vi "Temperature control panel.vi"(8 "error in (no error)":errorcluster, 9 "Data Source (0:Kelvin)":u16(ring) items=["Kelvin", "Celsius", "Sensor Units"], 10 "Input (0:A)":u16(ring) items=["A", "B"], 11 "VISA resource name":refnum<visa-resource-name>="GPIB0::12::INSTR") -> (0 "error out":errorcluster, 2 "Sensor Data":dbl format="%.4f", 3 "VISA resource name out":refnum<visa-resource-name>)   [LabVIEW 2020]
doc: "Reads and returns a single sensor reading from the instrument."
uses:
  Instance           1 36Saved   Sensor Data (Single Reading) .vi
  Lake Shore 335/Lake Shore 335.lvlib
panel:
  in  "Temperature Interval":dbl
  out "Graph":dbl(graph)
  in  "On/Off":bool
  in  "Range (0:Off)":u16(ring) items=["Off", "Low (On)", "Medium", "High"]
  in  "Manual Output (0.00 %)":dbl format="%.2f"
  in  "Heater Output (1:1)":u16(ring)=1 items=["1"=1, "2"=2]
  out "error out 4":errorcluster
  out "VISA resource name out 4":refnum<visa-resource-name>
  in  "error in (no error) 4":errorcluster
  in  "Setpoint start":bool
  in  "error in (no error) 3":errorcluster
  out "VISA resource name out 3":refnum<visa-resource-name>
  out "error out 3":errorcluster
  out "Setpoint":dbl format="%.4f"
  in  "Output (1:1)":u16(ring)=1 items=["1"=1, "2"=2]
  in  "error in (no error) 2":errorcluster
  out "VISA resource name out 2":refnum<visa-resource-name>
  out "error out 2":errorcluster
  in  "Output's Control Loop (1:1)":u16(ring)=1 items=["1"=1, "2"=2]
  in  "Setpoint (0.0000)":dbl format="%.4f"
  in  "Enable Setpoint Ramping (F: Off)":bool
  in  "Ramp Rate (0.0)":dbl=10.0 format="%.1f"
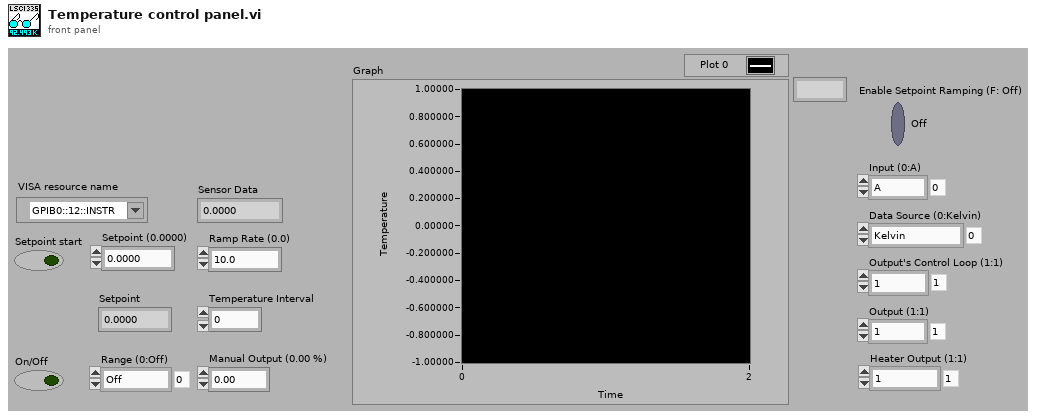
[diagram p1: front panel]
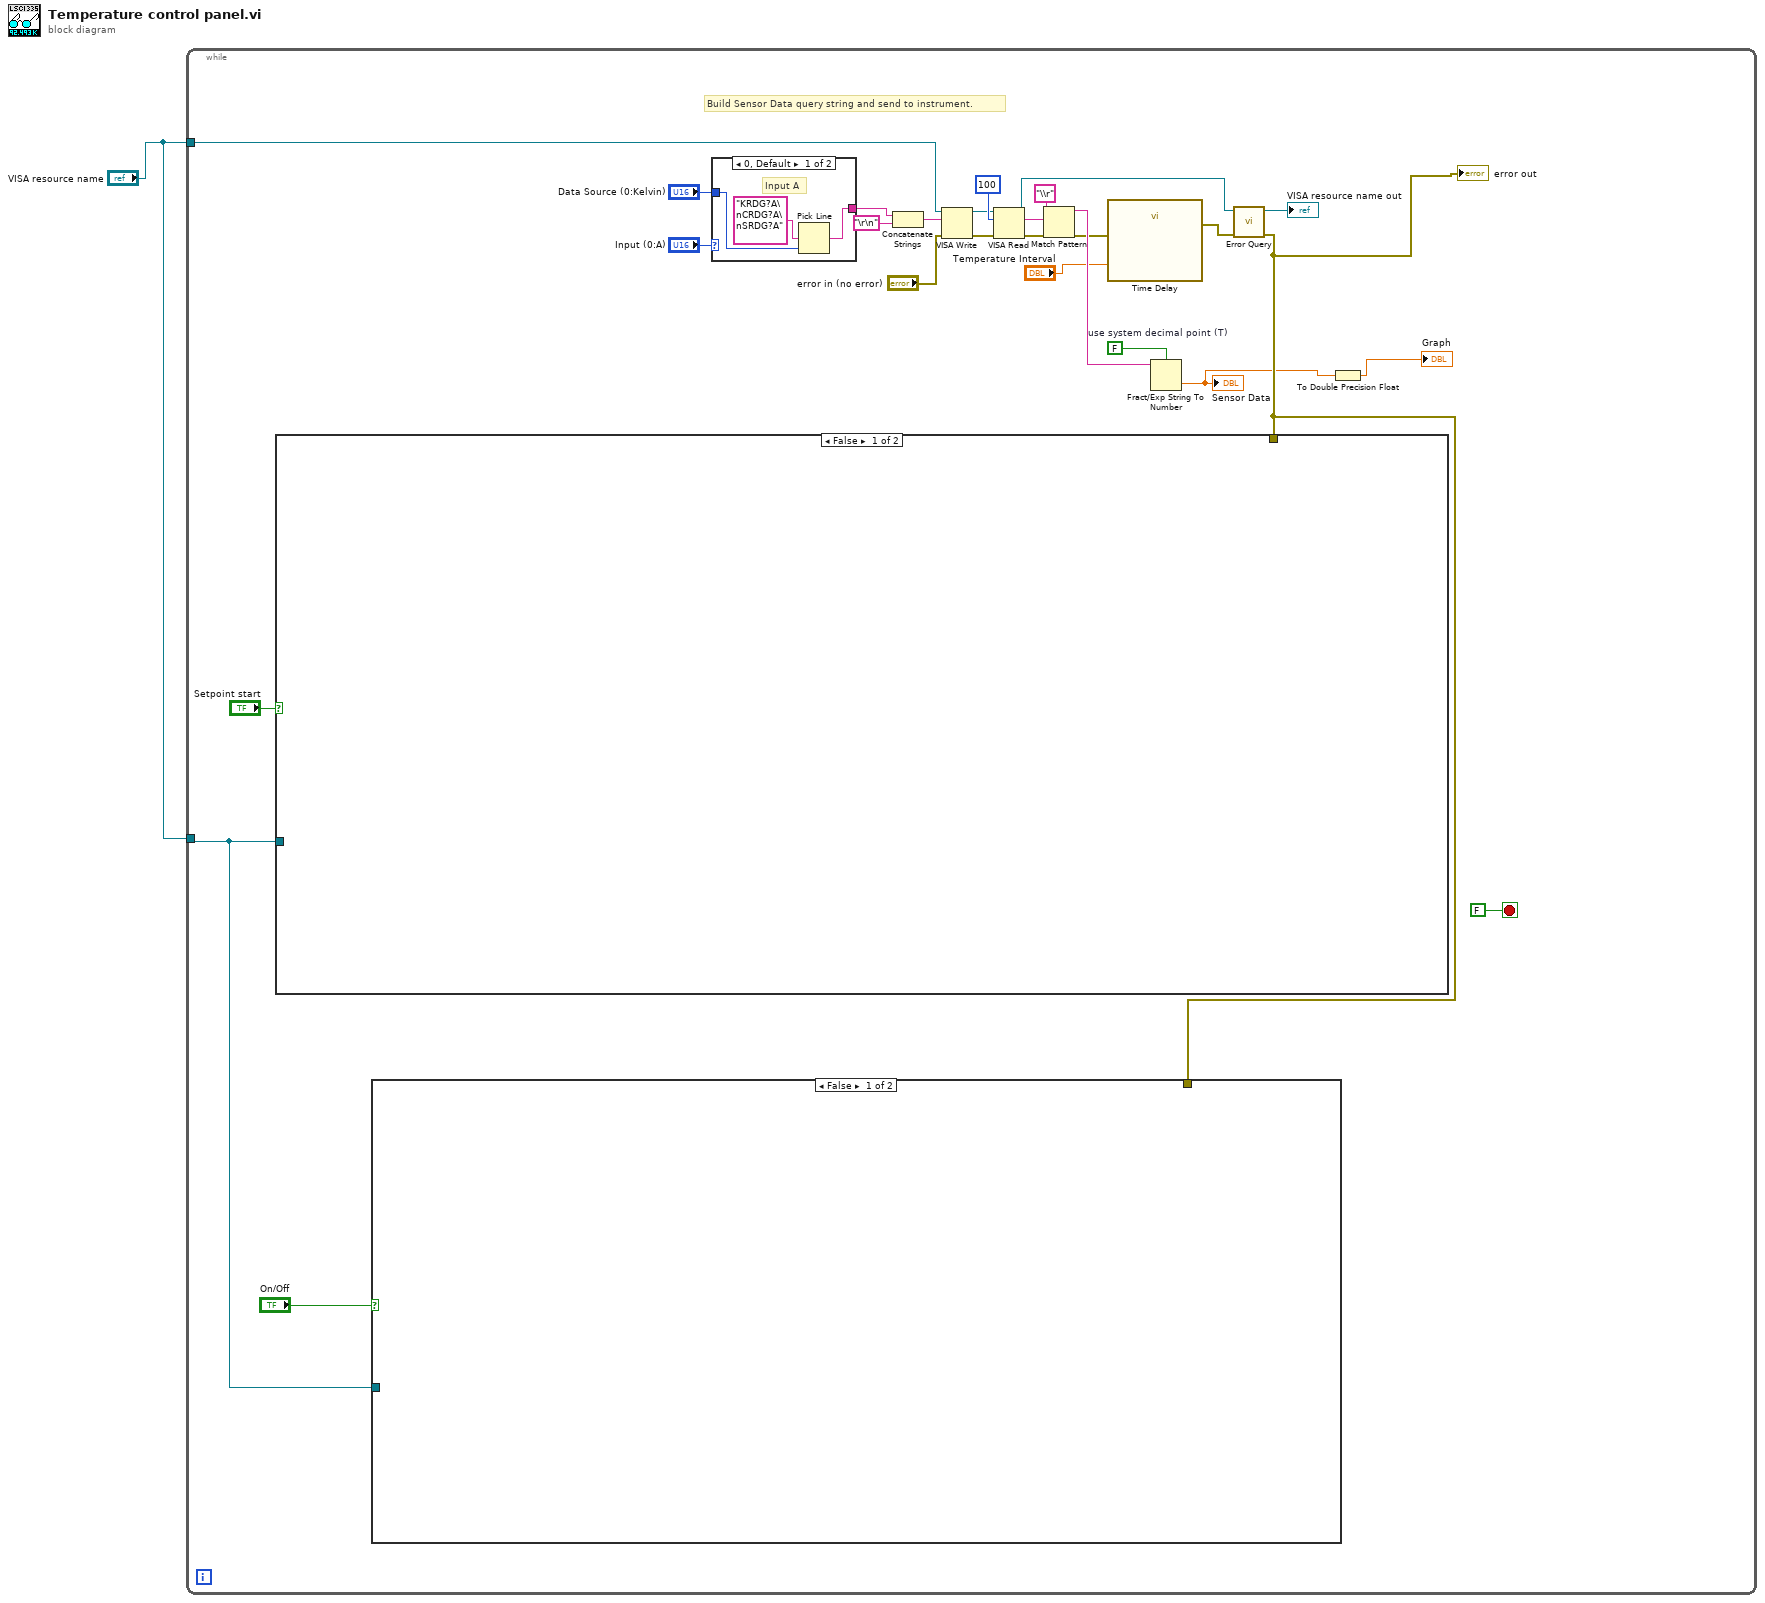
[diagram p0: block diagram]
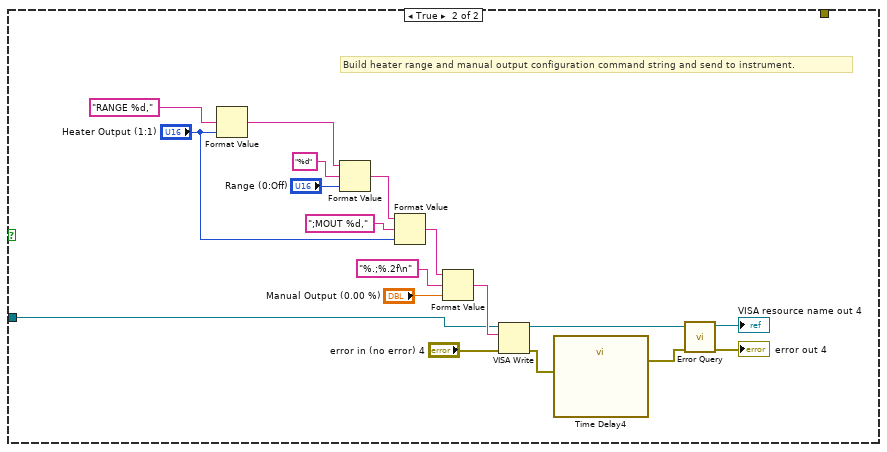
[diagram p2: hidden frame]
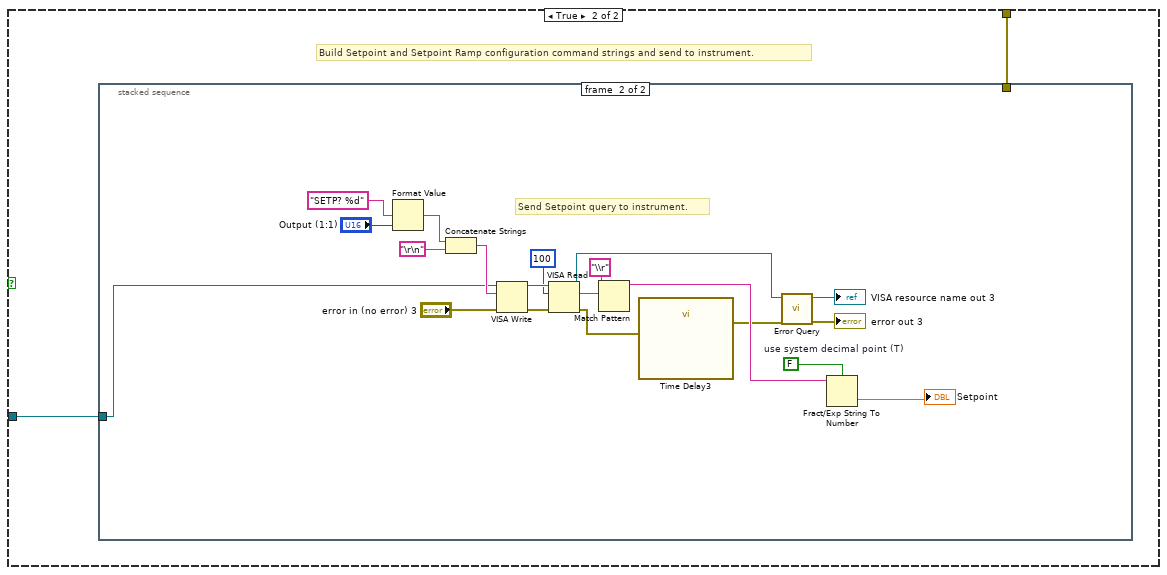
[diagram p3: hidden frame]
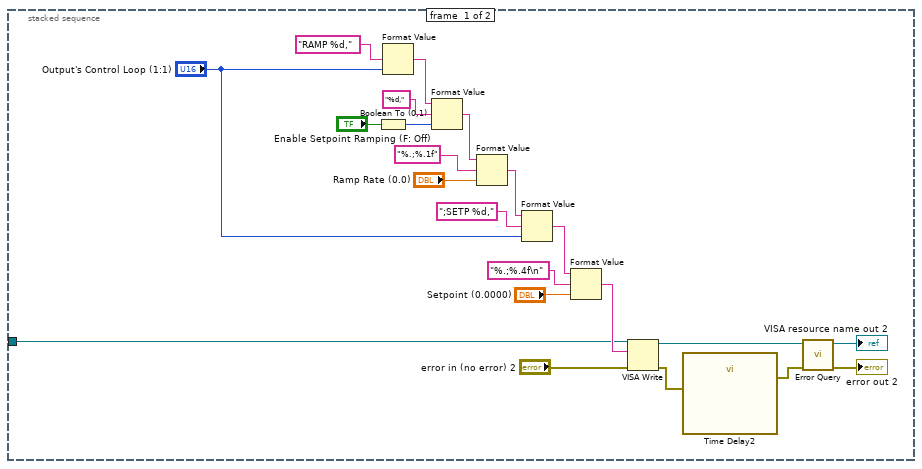
[diagram p4: hidden frame]
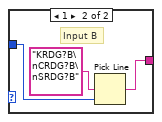
[diagram p5: hidden frame]
diagram:
  n1 = while {
    tunnel: "VISA resource name" -> [w8]
    tunnel: "VISA resource name" -> [w7]
    stop <- FALSE stop-if-true
    w19 = FALSE  # use system decimal point (T)
    # "Build Sensor Data query string and send to instrument."
    n2 = case shown="0, Default" "Input (0:A)" {
      tunnel: "Data Source (0:Kelvin)" -> [w91 w93]
      tunnel: [w90 w94] -> w11
      frame 0, Default {
        # "Input A"
        n3 = Pick Line(multi-line string="KRDG?A\nCRDG?A\nSRDG?A", line index=w91) -> (output string=w90:string)  [unwired: 1 in]
      }
      frame 1 {
        # "Input B"
        n4 = Pick Line(multi-line string="KRDG?B\nCRDG?B\nSRDG?B", line index=w93) -> (output string=w94:string)  [unwired: 1 in]
      }
    }
    n5 = Concatenate Strings(w11, "\r\n") -> (w12:string)
    n6 = VISA Write(VISA resource name=w8, write buffer=w12, error in (no error)="error in (no error)") -> (VISA resource name out=w21:refnum<visa-resource-name>, error out=w20:errorcluster)  [unwired: 1 out]
    n7 = VISA Read(VISA resource name=w21, byte count=100, error in (no error)=w20) -> (VISA resource name out=w25:refnum<visa-resource-name>, read buffer=w23:string, error out=w15:errorcluster)  [unwired: 1 out]
    n8 = Match Pattern(string=w23, regular expression="\\r") -> (before substring=w18:string)  [unwired: 1 in, 3 out]
    n9 = call "Time Delay"("error in (no error)"=w15, "Delay Time (s)"="Temperature Interval") -> ("error out"=w16:errorcluster)  [unwired: 9 in]
    n10 = Fract/Exp String To Number(use system decimal point (T)=w19, string=w18) -> (number=w3:dbl)  [unwired: 2 in, 1 out]
    "Sensor Data" <- w3
    n11 = call "Error Query.vi"("error in (no error)"=w16, "VISA resource name"=w25) -> ("error out"=w5:errorcluster, "VISA resource name out"=→"VISA resource name out":refnum<visa-resource-name>)  [unwired: 7 in, 1 out]
    "error out" <- w5
    n12 = case shown="False" "Setpoint start" {
      tunnel: w5 -> [_ w47]
      tunnel: w7 -> [_ w46]
      frame False {
      }
      frame True {
        # "Build Setpoint and Setpoint Ramp configuration command strings and send to instrument."
        n13 = stacked-sequence {
          tunnel: w47 -> [_ _]
          tunnel: w46 -> [w48 w70]
          frame #0 {
            n14 = Boolean To (0,1)(Boolean="Enable Setpoint Ramping (F: Off)") -> (0, 1=w53:i16)
            n15 = Format Value(format string="RAMP %d,", value (0)="Output's Control Loop (1:1)") -> (output string=w59:string)  [unwired: 1 in]
            n16 = Format Value(string ("")=w59, format string="%d,", value (0)=w53) -> (output string=w55:string)
            n17 = Format Value(string ("")=w55, format string="%.;%.1f", value (0)="Ramp Rate (0.0)") -> (output string=w51:string)
            n18 = Format Value(string ("")=w51, format string=";SETP %d,", value (0)="Output's Control Loop (1:1)") -> (output string=w60:string)
            n19 = Format Value(string ("")=w60, format string="%.;%.4f\n", value (0)="Setpoint (0.0000)") -> (output string=w62:string)
            n20 = VISA Write(VISA resource name=w48, write buffer=w62, error in (no error)="error in (no error) 2") -> (VISA resource name out=w69:refnum<visa-resource-name>, error out=w66:errorcluster)  [unwired: 1 out]
            n21 = call "Time Delay2"("error in (no error)"=w66) -> ("error out"=w65:errorcluster)  [unwired: 10 in]
            n22 = call "Error Query.vi"("error in (no error)"=w65, "VISA resource name"=w69) -> ("error out"=→"error out 2":errorcluster, "VISA resource name out"=→"VISA resource name out 2":refnum<visa-resource-name>)  [unwired: 7 in, 1 out]
          }
          frame #1 {
            w71 = FALSE  # use system decimal point (T)
            # "Send Setpoint query to instrument."
            n23 = Format Value(format string="SETP? %d", value (0)="Output (1:1)") -> (output string=w89:string)  [unwired: 1 in]
            n24 = Concatenate Strings(w89, "\r\n") -> (w81:string)
            n25 = VISA Write(VISA resource name=w70, write buffer=w81, error in (no error)="error in (no error) 3") -> (VISA resource name out=w77:refnum<visa-resource-name>, error out=w78:errorcluster)  [unwired: 1 out]
            n26 = VISA Read(VISA resource name=w77, byte count=100, error in (no error)=w78) -> (VISA resource name out=w84:refnum<visa-resource-name>, read buffer=w75:string, error out=w79:errorcluster)  [unwired: 1 out]
            n27 = Match Pattern(string=w75, regular expression="\\r") -> (before substring=w86:string)  [unwired: 1 in, 3 out]
            n28 = call "Time Delay3"("error in (no error)"=w79) -> ("error out"=w83:errorcluster)  [unwired: 10 in]
            n29 = call "Error Query.vi"("error in (no error)"=w83, "VISA resource name"=w84) -> ("error out"=→"error out 3":errorcluster, "VISA resource name out"=→"VISA resource name out 3":refnum<visa-resource-name>)  [unwired: 7 in, 1 out]
            n30 = Fract/Exp String To Number(use system decimal point (T)=w71, string=w86) -> (number=→"Setpoint":dbl)  [unwired: 2 in, 1 out]
          }
        }
      }
    }
    n31 = case shown="False" "On/Off" {
      tunnel: w7 -> [_ w28]
      tunnel: w5 -> [_ _]
      frame False {
      }
      frame True {
        # "Build heater range and manual output configuration command string and send to instrument."
        n32 = Format Value(format string="RANGE %d,", value (0)="Heater Output (1:1)") -> (output string=w41:string)  [unwired: 1 in]
        n33 = Format Value(string ("")=w41, format string="%d", value (0)="Range (0:Off)") -> (output string=w40:string)
        n34 = Format Value(string ("")=w40, format string=";MOUT %d,", value (0)="Heater Output (1:1)") -> (output string=w29:string)
        n35 = Format Value(string ("")=w29, format string="%.;%.2f\n", value (0)="Manual Output (0.00 %)") -> (output string=w35:string)
        n36 = VISA Write(VISA resource name=w28, write buffer=w35, error in (no error)="error in (no error) 4") -> (VISA resource name out=w36:refnum<visa-resource-name>, error out=w38:errorcluster)  [unwired: 1 out]
        n37 = call "Time Delay4"("error in (no error)"=w38) -> ("error out"=w37:errorcluster)  [unwired: 10 in]
        n38 = call "Error Query.vi"("error in (no error)"=w37, "VISA resource name"=w36) -> ("error out"=→"error out 4":errorcluster, "VISA resource name out"=→"VISA resource name out 4":refnum<visa-resource-name>)  [unwired: 7 in, 1 out]
      }
    }
    n39 = To Double Precision Float(number=w3) -> (double precision float=→"Graph":dbl)
  }
